vi "timedelay.vi"() -> ()   [LabVIEW 2015]
uses:
  BERTTA.dll
panel:
  out "element 3":i32
  out "element 2":i32
  out "element":i32
  in  "delay":i32
  in  "start":i32
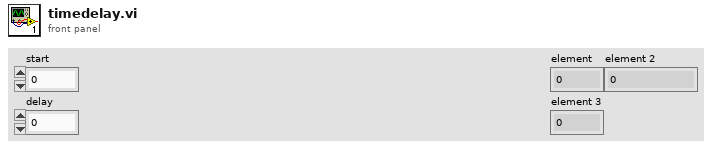
[diagram p1: front panel]
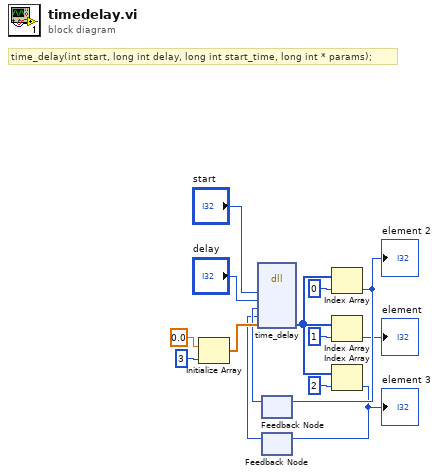
[diagram p0: block diagram]
diagram:
  # "time_delay(int start, long int delay, long int start_time, long int * params);"
  n1 = Initialize Array(0.0 ("element"), 3 ("dimension size")) -> (w14:dbl[])
  n2 = feedback #1() -> (w9:i32)  [unwired: 1 in]
  n3 = feedback #2() -> (w1:i32)  [unwired: 1 in]
  n4 = dll-call lib="C:/Users/shresplab/OneDrive - Kemira Oyj/Documents/Visual Studio 2017/Projects/Bertta/BERTTA/x64/Debug/BERTTA.dll" fn="time_delay"("start"="start", "delay"="delay", "start_time"=w9, "start_"=w1, "params"=w14) -> ("params"=w3:i32[])  [unwired: 8 in, 2 out]
  n5 = Index Array(array=w3, index=0) -> (element=w10:i32)
  "element 2" <- w10
  n6 = feedback-in #1(w10) -> ()
  n7 = Index Array(array=w3, index=1) -> (element=→"element":i32)
  n8 = Index Array(array=w3, index=2) -> (element=w2:i32)
  "element 3" <- w2
  n9 = feedback-in #2(w2) -> ()
